vi "Generated_Regression.vi"(8 "error in (no error)":errorcluster caption="entrée d'erreur (pas d'erreur)", 11 "make_regression":T2={"n_samples"=100, "n_features"=100, "n_informative"=10, "n_targets"=1, "bias"=0.0, "effective_rank"="None", "tail_strength"=0.5, "noise"=0.0, "shuffle"=TRUE, "random_state"=-1, "Returns"="X"} {"tail_strength" min=0.0 max=1.0; "n_targets" min=1; "n_features" min=1; "n_samples" min=1}) -> (0 "error out":errorcluster, 3 "Data":T1)   [LabVIEW 2020]
doc: "Generate a random regression problem.\n\nThe input set can either be well conditioned (by default) or have a low rank-fat tail singular profile. See make_low_rank_matrix for more details.\n\nThe output is generated by applying a (potentially biased) random linear regression model with n_informative nonzero regressors to the previously generated input and some gaussian centered noise with some adjustable scale.\n\n\n\nParameters :\n\n- n_samples : int, optional (default=100)\nThe number of samples.\n\n- n_features : int, optional (default=100)\nThe number of features.\n\n- n_informative : int, optional (default=10)\nThe number of informative features, i.e., the number of features used to build the linear model used to generate the output.\n\n- n_targets : int, optional (default=1)\nThe number of regression targets, i.e., the dimension of the y output vector associated with a sample. By default, the output is a scalar.\n\n- bias : float, optional (default=0.0)\nThe bias term in the underlying linear model.\n\n- effective_rank : int or None, optional (default=None)\nif not None:\nThe approximate number of singular vectors required to explain most of the input data by linear combinations. Using this kind of singular spectrum in the input allows the generator to reproduce the correlations often observed in practice.\n\nif None:\nThe input set is well conditioned, centered and gaussian with unit variance.\n\n- tail_strength : float between 0.0 and 1.0, optional (default=0.5)\nThe relative importance of the fat noisy tail of the singular values profile if effective_rank is not None.\n\n- noise : float, optional (default=0.0)\nThe standard deviation of the gaussian noise applied to the output.\n\n- shuffle : boolean, optional (default=True)\nShuffle the samples and the features.\n\n- random_state : int, RandomState instance, default=None=-1\nDetermines random number generation for dataset creation. Pass an int for reproducible output across multiple function calls. See Glossary.\n\nReturns :\n\n- X : array of shape [n_samples, n_features]\nThe input samples.\n\n- y : array of shape [n_samples] or [n_samples, n_targets]\nThe output values.\n\n- coef : array of shape [n_features] or [n_features, n_targets], optional\nThe coefficient of the underlying linear model. It is returned only if coef is True."
uses:
  Regression.lvclass
panel:
  out "Regression.lvclass":refnum<class "Regression.lvclass">
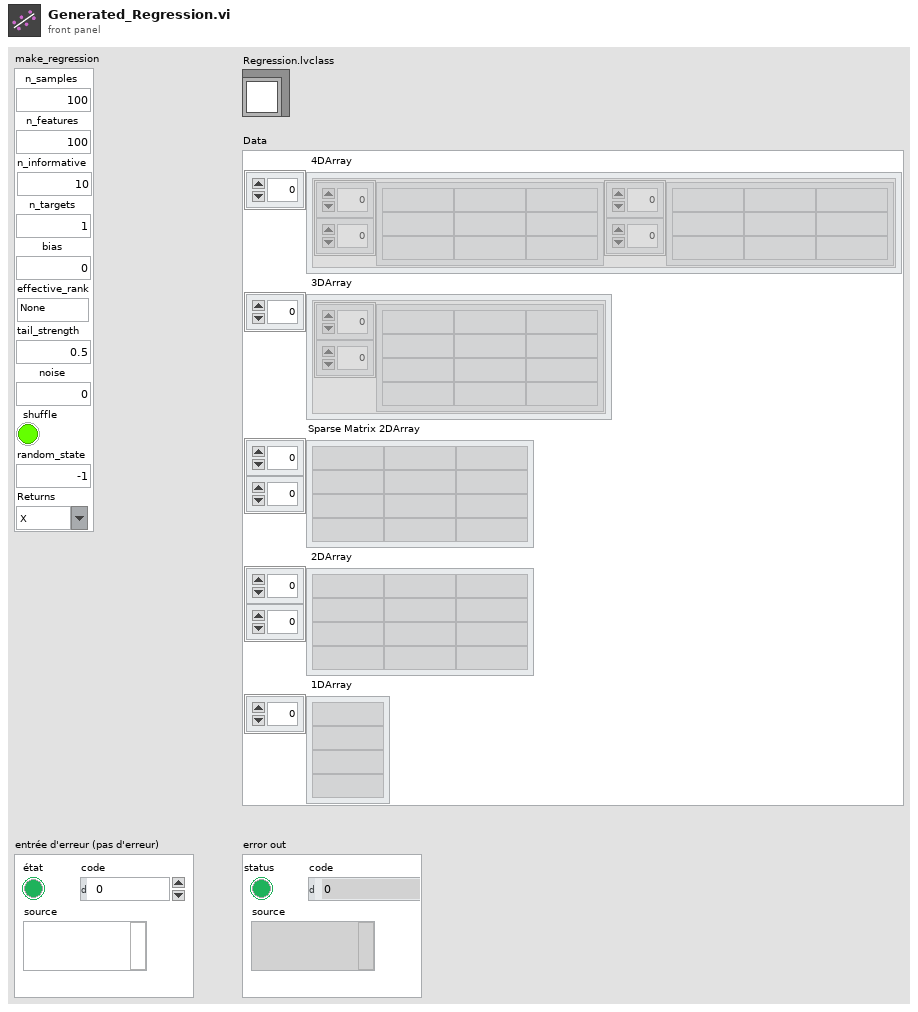
[diagram p1: front panel]
types:
  T1 = cluster{" 4DArray":cluster{"1":string[][], "2":string[][]}[], " 3DArray":cluster{"Tableau":string[][]}[], "Sparse Matrix 2DArray":string[][], " 2DArray":string[][], " 1DArray":string[]}
  T2 = cluster{"n_samples":u32, "n_features":u32, "n_informative":u32, "n_targets":u32, "bias":dbl, "effective_rank":string, "tail_strength":dbl, "noise":dbl, "shuffle":bool, "random_state":i32, "Returns":string}
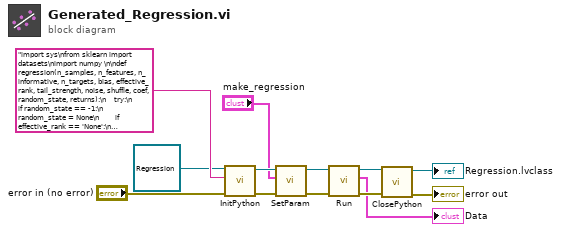
[diagram p0: block diagram]
diagram:
  n1 = call-dynamic "InitPython.vi"("error in (no error)"="error in (no error)", "Python Instruction"="import sys\nfrom sklearn import datasets\nimport numpy \n\ndef regression(n_samples, n_features, n_informative, n_targets, bias, effective_rank, tail_strength, noise, shuffle, coef, random_state, returns):\n    try:\n        if random_state == -1:\n            random_state = None\n        if effective_rank == 'None':\n            effective_rank = None\n        else: \n            effective_rank = eval(effective_rank)\n        X, y, coef = datasets.make_regression(n_samples, n_features, n_informative, n_targets, bias, effective_rank, tail_strength, noise, shuffle, coef, random_state)\n        if returns == 'X':\n            dataX = X.tolist()\n            return str(dataX) \n        elif returns == 'Y':\n            datay = y.tolist()\n            return str(datay)\n        else:\n            data_coef = coef.tolist()\n            return str(data_coef)\n    except:\n        erreur = sys.exc_info()\n        typerr = u\"%s\" % (erreur[0])\n        typerr = typerr[typerr.find(\"'\")+1:typerr.rfind(\"'\")]\n        msgerr = u\"%s\" % (erreur[1])\n        message = str('/!\\\\ {0} : {1}'. format(typerr,msgerr))\n        return message", "Scikit-learn en entrée"=refnum<class "Regression.lvclass"> refnum ("Regression.lvclass")) -> ("error out"=w9:errorcluster, "Scikit-learn en sortie"=w10:refnum<class "Regression.lvclass">)  [unwired: 7 in]
  n2 = call-dynamic "SetParam.vi"("error in (no error)"=w9, "make_regression"="make_regression", "Regression.lvclass"=w10) -> ("error out"=w6:errorcluster, "Regression.lvclass"=w7:refnum<class "Regression.lvclass">)  [unwired: 7 in]
  n3 = call-dynamic "Run.vi"("error in (no error)"=w6, "Regression.lvclass"=w7) -> ("error out"=w4:errorcluster, "Data"=→"Data":T1, "Regression.lvclass"=w5:refnum<class "Regression.lvclass">)  [unwired: 7 in]
  n4 = call-dynamic "ClosePython.vi"("error in (no error)"=w4, "Scikit-learn en entrée"=w5) -> ("error out"=→"error out":errorcluster, "Scikit-learn en sortie"=→"Regression.lvclass":refnum<class "Regression.lvclass">)  [unwired: 8 in]
